vi "Balance_Sweep_Client.vi"(5 "Stop Angle":dbl) -> (1 "Data Out":string)   [LabVIEW 2011]
uses:
  OGI_Server/ATE_Balance_Data.ctl
  <vilib>/Platform/TimedLoop/XDataNode/timing_clust.ctl
  <vilib>/Platform/TimedLoop/XDataNode/nitl_modes.ctl
  <vilib>/Platform/TimedLoop/XDataNode/wakeup.ctl
  Globals/Trav_pos_global.vi
  <vilib>/Platform/TimedLoop/XDataNode/XDataNode.xnode
  <vilib>/Platform/TimedLoop/XDataNode/XDNodeRunTimeDep.lvlib
panel:
  out "Live Angle":dbl
  out "Target Angle":dbl
  out "Balance Data Ref":refnum<k21>
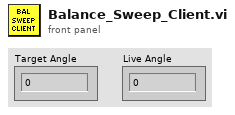
[diagram p1: front panel]
types:
  T1 = typedef "XDNodeRunTimeDep.lvlib/timing_clust.ctl" = cluster{"Expected End [f-1]":u64, "Actual End [f-1]":u64, "Finished Late? [f-1]":bool, "Expected End [i-1]":u64, "Actual End [i-1]":u64, "Finished Late? [i-1]":bool, "Expected Start [i]":u64, "Actual Start [i]":u64, "Expected Start [f]":u64, "Actual Start [f]":u64, "Source Name":string, "Structure Name":string, "Period":i64, "Deadline":i64, "Offset":i64, "Start":i64, "Priority":i32, "Timeout":i32, "Mode":T2, "Wakeup Reason":T3, "Error":errorcluster, "Source Type":string, "Secondary Source Type":string, "Global End Time":u64, "Global Start Time":u64, "Frame Duration":u64, "Iteration Duration":u64, "Assigned CPU":i32, "I/O Scan Engine Mode":u32}
  T2 = typedef "XDNodeRunTimeDep.lvlib/nitl_modes.ctl" = enum32{"No Change", "Process missed periods, maintain original phase", "Discard missed periods, maintain original phase", "Process missed periods, ignore original phase", "Discard missed periods, ignore original phase"}
  T3 = typedef "XDNodeRunTimeDep.lvlib/wakeup.ctl" = enum32{"Normal", "Aborted", "Asynchronous wakeup", "Timing source error", "Timed loop error", "Timeout"}
  T4 = enum16{"big-endian, network order", "native, host order", "little-endian"}
  T5 = typedef "ATE_Balance_Data.ctl" = cluster{"%Lift":dbl, "Lift":dbl, "%Pitch":dbl, "Pitch":dbl, "%Drag":dbl, "Drag":dbl, "%Side":dbl, "Side":dbl, "%Yaw":dbl, "Yaw":dbl, "%Roll":dbl, "Roll":dbl}
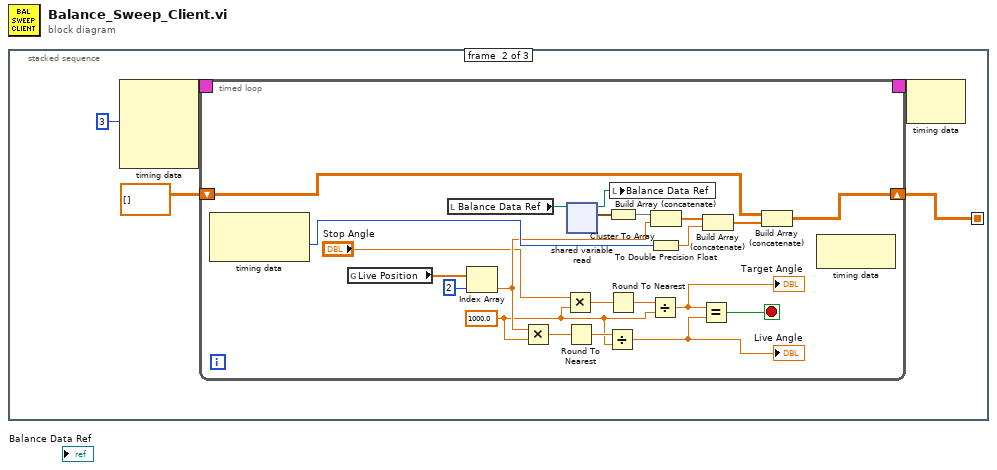
[diagram p0: block diagram]
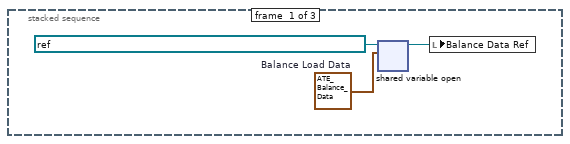
[diagram p2: hidden frame]
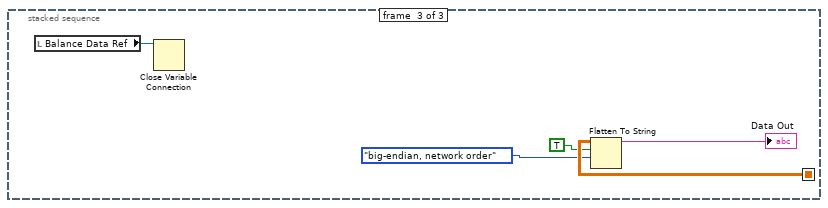
[diagram p3: hidden frame]
diagram:
  n1 = stacked-sequence {
    seq-local: [_ w5 _] -> [_ _ w41]
    frame #0 {
      w2 = T5 {"%Lift"=0.0, "Lift"=0.0, "%Pitch"=0.0, "Pitch"=0.0, "%Drag"=0.0, "Drag"=0.0, "%Side"=0.0, "Side"=0.0, "%Yaw"=0.0, "Yaw"=0.0, "%Roll"=0.0, "Roll"=0.0}  # Balance Load Data
      n2 = shared-variable-open(refnum<k21> "ni.var.psp://192.168.8.2/ATE_Shared_Variables/Balance_Data" ("shared variable refnum in"), w2) -> (w1:refnum<k21>)  [unwired: 2 in, 1 out]
      n3 = local write "Balance Data Ref"(w1) -> ()
    }
    frame #1 {
      n4 = node-c288(i64 3 ("Period")) -> (w8:T1)  [unwired: 3 in]
      n5 = timed-loop {
        timing: w8 -> [_]
        timing-out: [_] -> w7
        shift-right: [w22] -> w5
        shift-left: dbl[][] [] -> [w21]
        stop <- w20 stop-if-true
        w12 = 1000.0 ("y")
        n6 = node-c288() -> (w24:i64)  [unwired: 1 in, 1 out]
        n7 = global read "Trav_pos_global.vi" "Live Position"() -> (w28:dbl[])
        n8 = local read "Balance Data Ref"() -> (w30:refnum<k21>)
        n9 = Index Array(array=w28, index=2) -> (element=w16:dbl)
        n10 = Multiply(x=w16, y=w12) -> (x*y=w13:dbl)
        n11 = Multiply(x="Stop Angle", y=w12) -> (x*y=w19:dbl)
        n12 = Round To Nearest(number=w13) -> (nearest integer value=w14:dbl)
        n13 = shared-variable-read(w30) -> (w29:refnum<k21>, w26:T5)  [unwired: 1 in, 2 out]
        n14 = Divide(x=w14, y=w12) -> (x/y=w15:dbl)
        "Live Angle" <- w15
        n15 = Cluster To Array(cluster=w26) -> (array=w25:dbl[])
        n16 = Round To Nearest(number=w19) -> (nearest integer value=w18:dbl)
        n17 = local write "Balance Data Ref"(w29) -> ()
        n18 = Divide(x=w18, y=w12) -> (x/y=w17:dbl)
        "Target Angle" <- w17
        n19 = Build Array (concatenate)(w25, w16) -> (w10:dbl[])
        n20 = To Double Precision Float(number=w24) -> (double precision float=w11:dbl)
        n21 = Equal?(x=w17, y=w15) -> (x = y?=w20:bool)
        n22 = Build Array (concatenate)(w10, w11) -> (w23:dbl[])
        n23 = Build Array (concatenate)(w21, w23) -> (w22:dbl[][])
        n24 = node-c288() -> ()  [unwired: 1 in, 1 out]
      }
      n25 = node-c288(w7) -> ()  [unwired: 1 out]
    }
    frame #2 {
      n26 = local read "Balance Data Ref"() -> (w42:refnum<k21>)
      n27 = Close Variable Connection(11:w42) -> ()  [unwired: 1 in, 1 out]
      n28 = Flatten To String(anything=w41, prepend array or string size? (T)=TRUE, byte order (0:big-endian, network order)=T4."big-endian, network order") -> (data string=→"Data Out":string)  [unwired: 1 in, 2 out]
    }
  }
